vi "tlc_Play_Update Cue.vi"(5 "Target Time":dbl, 7 "Elapsed Time":dbl, 8 "error in":errorcluster, 9 "Cue States":T1[][](array[typedef]), 10 "Cue Input":T2 {"Channels"."Intensity" min=0.0 max=100.0 step=1.0 format="%#.0f"}) -> (0 "error out":errorcluster, 2 "Cue Output":T2 {"Channels"."Intensity" min=0.0 max=100.0 step=1.0 format="%#.0f"})   [LabVIEW 2010]
doc: "This VI will increase or decrease the intensity of a channel in the Theatre Light Controller."
uses:
  Controls/tlc_Cue_Information.ctl
  Controls/channel.ctl
  Controls/Cue State.ctl
  Controls/tlc_User Interface Data Type.ctl
  Modules/Hardware/tlc_Hardware_Command Control.ctl
panel:
  # "Input"
  # "Output"
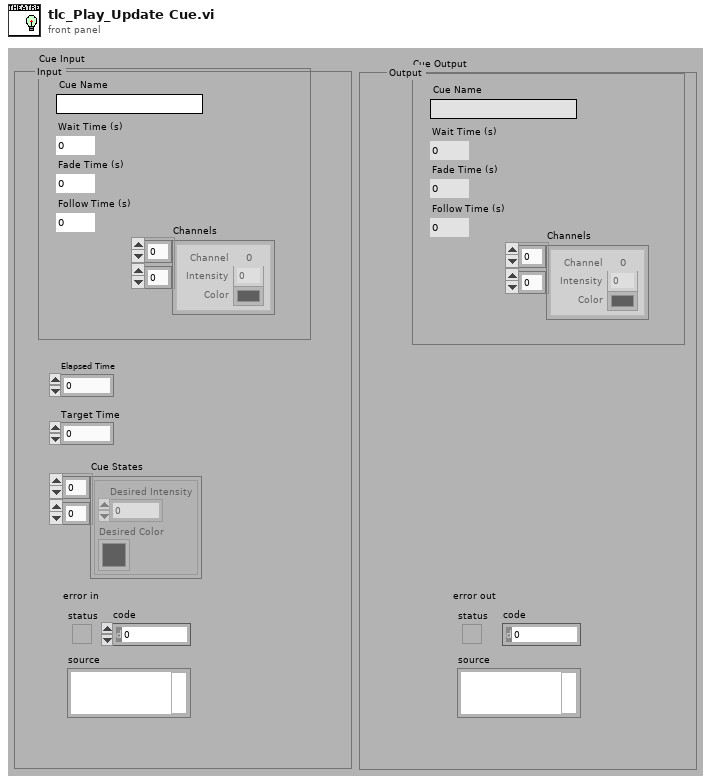
[diagram p1: front panel]
types:
  T1 = typedef "Cue State.ctl" = cluster{"Desired Intensity":dbl, "Desired Color":u32}
  T2 = typedef "tlc_Cue_Information.ctl" = cluster{"Cue Name":string, "Wait Time (s)":u32, "Fade Time (s)":u32, "Follow Time (s)":u32, "Channels":T3[][]}
  T3 = typedef "channel.ctl" = cluster{"Intensity":dbl, " Color":u32, "Channel":i32}
  T4 = typedef "tlc_User Interface Data Type.ctl" = enum16{"Initialize", "Initialize Front Panel", "Update Front Panel Channels", "Select Cue in Cue List", "Enable/Disable Front Panel Controls", "Update Cue List", "Stop"}
  T5 = typedef "tlc_Hardware_Command Control.ctl" = enum16{"Initialize", "Write", "Shutdown"}
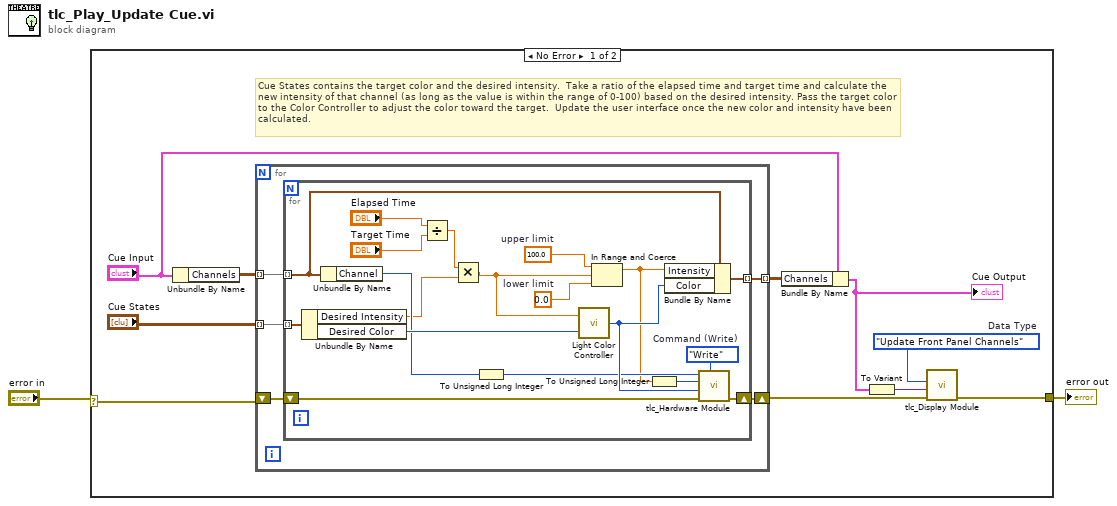
[diagram p0: block diagram]
diagram:
  n1 = case shown="No Error" "error in" {
    selector: "error in" -> [w6 w37]
    tunnel: [w5 w37] -> w1
    frame No Error {
      w9 = tlc_User_Interface_Data_Type."Update Front Panel Channels"  # Data Type
      # "Cue States contains the target color and the desired intensity.  Take a ratio of the elapsed time and target time and calculate the new intensity of that channel (as long as the value is within the range of 0-100) based on the desired intensity. Pass the target color to the Color Controller to adjust the color toward the target.  Update the user interface once the new color and intensity have been calculated."
      n2 = Unbundle By Name("Cue Input") -> ("Channels"=w11:T3[][])
      n3 = for {
        tunnel: w11 -> [w17] mode=indexing
        tunnel: [w16] -> w12 mode=indexing
        shift-right: [w14] -> w10
        shift-left: w6 -> [w15]
        tunnel: "Cue States" -> [w13] mode=indexing
        n4 = for {
          tunnel: w17 -> [w36] mode=indexing
          tunnel: [w35] -> w16 mode=indexing
          shift-right: [w33] -> w14
          shift-left: w15 -> [w34]
          tunnel: w13 -> [w32] mode=indexing
          w27 = 0.0  # lower limit
          w28 = 100.0  # upper limit
          w30 = tlc_Hardware_Command_Control."Write"  # Command (Write)
          n5 = Unbundle By Name(w32) -> ("Desired Intensity"=w18:dbl, "Desired Color"=w31:u32)
          n6 = Unbundle By Name(w36) -> ("Channel"=w25:i32)
          n7 = Divide(x="Elapsed Time", y="Target Time") -> (x/y=w19:dbl)
          n8 = Multiply(x=w19, y=w18) -> (x*y=w20:dbl)
          n9 = To Unsigned Long Integer(number=w25) -> (unsigned 32bit integer=w26:u32)
          n10 = call "Light Color Controller.vi"("Input Color"=w31, "Intensity"=w20) -> ("Output Color"=w29:u32)
          n11 = In Range and Coerce(upper limit=w28, x=w20, lower limit=w27) -> (coerced(x)=w24:dbl)  [unwired: 1 out]
          n12 = To Unsigned Long Integer(number=w24) -> (unsigned 32bit integer=w23:u32)
          n13 = Bundle By Name(cluster=w36, "Intensity"=w24, "Color"=w29) -> (w35:T3)
          n14 = call "tlc_Hardware Module.vi"("Command (Write)"=w30, "error in (no error)"=w34, "Color"=w29, "Intensity"=w23, "Channel"=w26) -> ("error out"=w33:errorcluster)  [unwired: 6 in]
        }
      }
      n15 = Bundle By Name(cluster="Cue Input", "Channels"=w12) -> (w4:T2)
      "Cue Output" <- w4
      n16 = To Variant(anything=w4) -> (Variant=w3:variant)
      n17 = call "tlc_Display Module.vi"("error in (no error)"=w10, "Data"=w3, "Data Type"=w9) -> ("error out"=w5:errorcluster)  [unwired: 8 in]
    }
    frame Error {
    }
  }
  "error out" <- w1
